vi "Get Controls in Cluster.vi"(5 "Owner Labels":string[](array[string]), 7 "Owner Classes":string[](array[string]), 8 "error in (no error)":errorcluster, 9 "Owning Pane":refnum<vi>, 10 "Control Map":map{string, T1[]}(c390), 11 "Cluster Ref":refnum<vi>) -> (0 "error out":errorcluster, 2 "Control Map out":map{string, T1[]}(c390), 3 "Cluster Ref out":refnum<vi>)   [LabVIEW 2020, in "MacroAssert.lvlib"]
doc: "Gets all control references within <B>Cluster Ref</B> recursively by checking it for nested clusters, getting any controls in them, and so on."
uses:
  MacroAssert.lvlib
  CTLs/Control Map Control Data.ctl
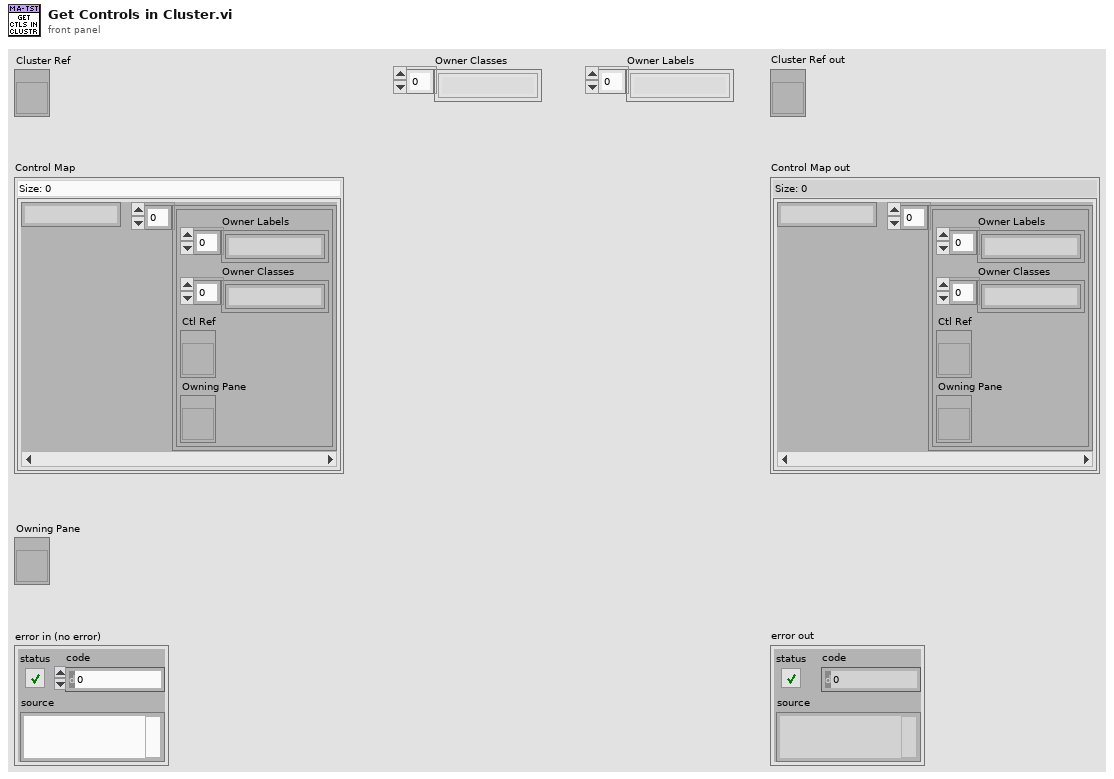
[diagram p1: front panel]
types:
  T1 = typedef "MacroAssert.lvlib/Control Map Control Data.ctl" = cluster{"Owner Labels":string[], "Owner Classes":string[], "Ctl Ref":refnum<vi>, "Owning Pane":refnum<vi>}
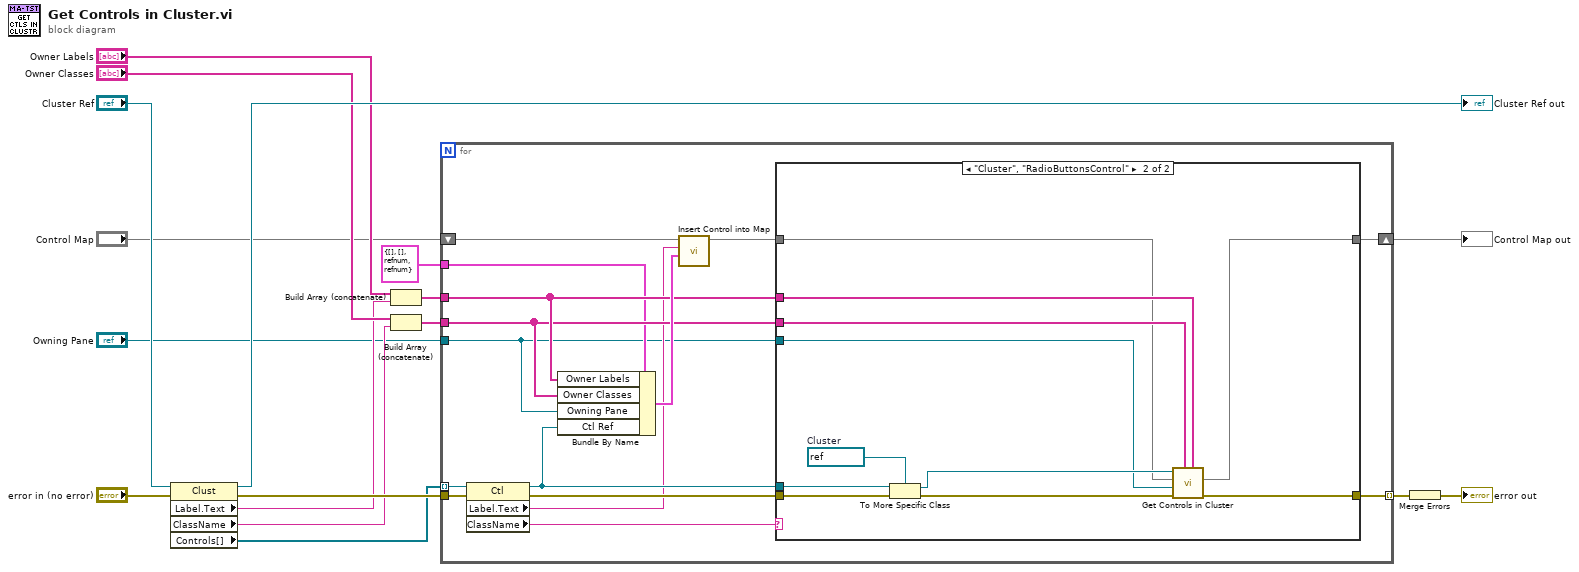
[diagram p0: block diagram]
diagram:
  n1 = property class="Clust"(reference="Cluster Ref", error in="error in (no error)") -> (reference out=→"Cluster Ref out":refnum<vi>, error out=w15:errorcluster, "Label.Text"=w8:string, "ClassName"=w7:string, "Controls[]"=w11:refnum<vi>[])
  n2 = Build Array (concatenate)("Owner Labels", w8) -> (w6:string[])
  n3 = Build Array (concatenate)("Owner Classes", w7) -> (w5:string[])
  n4 = for {
    tunnel: [w32] -> w12 mode=indexing
    tunnel: w15 -> [w30]
    tunnel: w11 -> [w29] mode=indexing
    tunnel: w6 -> [w24]
    tunnel: w5 -> [w23]
    shift-right: [w18] -> w1
    shift-left: "Control Map" -> [w26]
    tunnel: "Owning Pane" -> [w19]
    tunnel: T1 {"Owner Labels"=[], "Owner Classes"=[], "Ctl Ref"=refnum, "Owning Pane"=refnum} ("Ctl Data") -> [w22]
    n5 = property class="Ctl"(reference=w29, error in=w30) -> (reference out=w25:refnum<vi>, error out=w31:errorcluster, "Label.Text"=w21:string, "ClassName"=w28:string)
    n6 = Bundle By Name(cluster=w22, "Owner Labels"=w24, "Owner Classes"=w23, "Owning Pane"=w19, "Ctl Ref"=w25) -> (w27:T1)
    n7 = call "Insert Control into Map.vi"("Ctl Data"=w27, "Name"=w21, "Control Map"=w26) -> ("Control Map out"=w20:map{string, T1[]})  [unwired: 8 in]
    n8 = case shown="\"Cluster\", \"RadioButtonsControl\"" w28 {
      tunnel: [w34 w43] -> w32
      tunnel: w25 -> [_ w41]
      tunnel: w31 -> [w34 w45]
      tunnel: w24 -> [_ w38]
      tunnel: w23 -> [_ w39]
      tunnel: w20 -> [w33 w37]
      tunnel: w19 -> [_ w36]
      tunnel: [w33 w35] -> w18
      frame Default {
      }
      frame "Cluster", "RadioButtonsControl" {
        w42 = refnum<vi> refnum  # Cluster
        n9 = To More Specific Class(target class=w42, reference=w41, error in=w45) -> (specific class reference=w40:refnum<vi>, error out=w44:errorcluster)
        n10 = call "Get Controls in Cluster.vi"("Owner Labels"=w38, "Owner Classes"=w39, "error in (no error)"=w44, "Owning Pane"=w36, "Control Map"=w37, "Cluster Ref"=w40) -> ("error out"=w43:errorcluster, "Control Map out"=w35:map{string, T1[]})  [unwired: 3 in, 1 out]
      }
    }
  }
  "Control Map out" <- w1
  n11 = Merge Errors(w12) -> (→"error out":errorcluster)
